vi "Run.vi"(8 "error in (no error)":errorcluster caption="entrée d'erreur (pas d'erreur)", 11 "Biclusters.lvclass":refnum<class "Biclusters.lvclass">) -> (0 "error out":errorcluster caption="sortie d'erreur", 2 "Data":T1, 3 "Biclusters.lvclass":refnum<class "Biclusters.lvclass">)   [LabVIEW 2020, in "Biclusters.lvclass"]
doc: "Returns : \n\nX : array of shape shape\n The generated array.\n\nrows : array of shape (n_clusters, X.shape[0],)\nThe indicators for cluster membership of each row.\n\ncols : array of shape (n_clusters, X.shape[1],)\nThe indicators for cluster membership of each column."
uses:
  Biclusters.lvclass
  Biclusters.lvclass/Biclusters.ctl
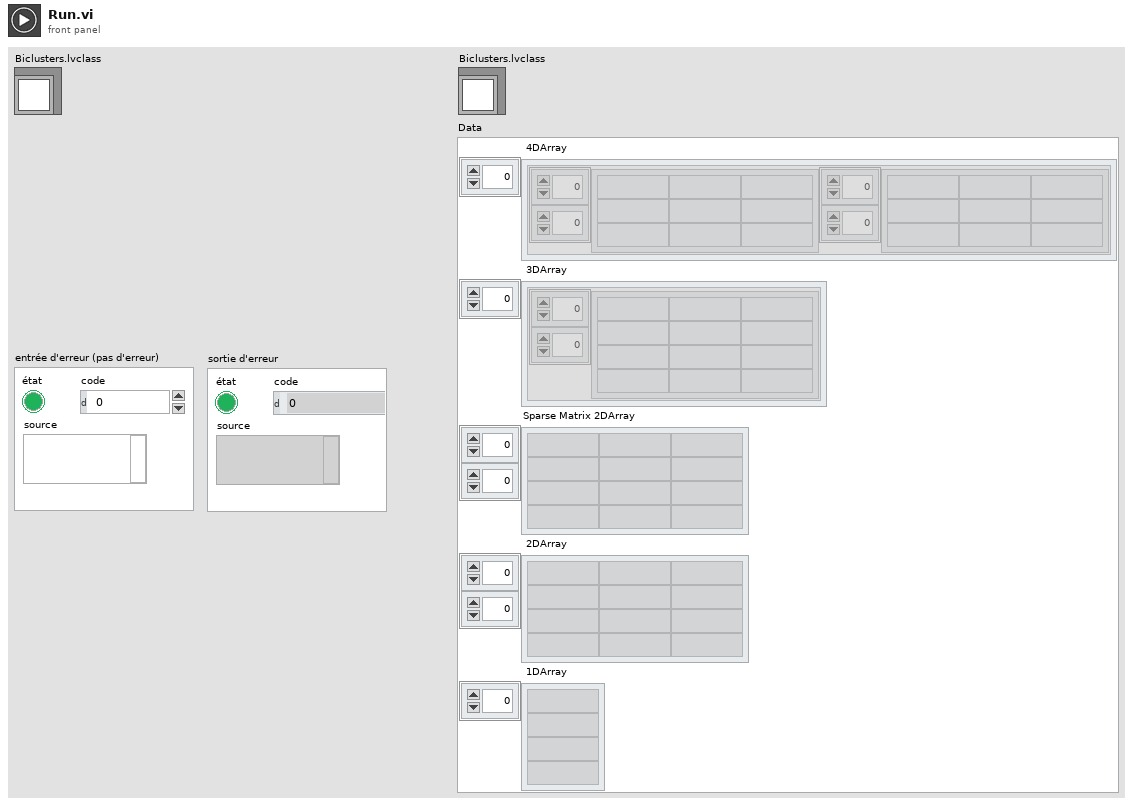
[diagram p1: front panel]
types:
  T1 = cluster{" 4DArray":cluster{"1":string[][], "2":string[][]}[], " 3DArray":cluster{"Tableau":string[][]}[], "Sparse Matrix 2DArray":string[][], " 2DArray":string[][], " 1DArray":string[]}
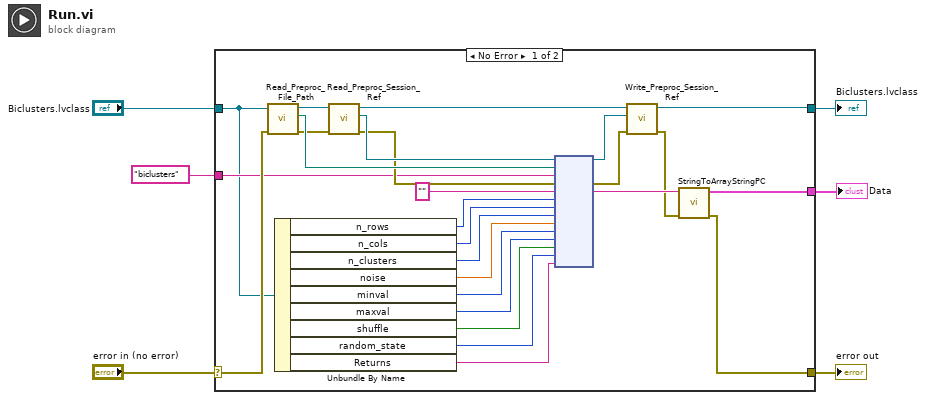
[diagram p0: block diagram]
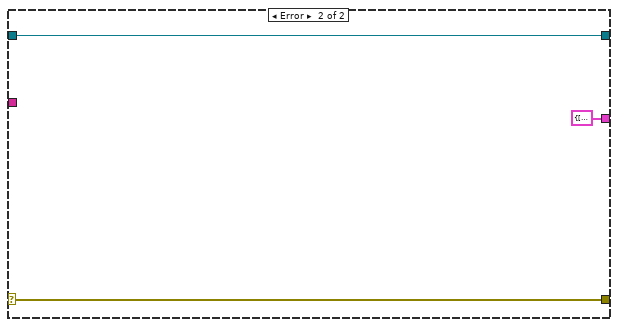
[diagram p2: hidden frame]
diagram:
  n1 = case shown="No Error" "error in (no error)" {
    selector: "error in (no error)" -> [w23 w35]
    tunnel: [w7 w35] -> w5
    tunnel: [w11 w34] -> w3
    tunnel: "Biclusters.lvclass" -> [w21 w34]
    tunnel: "biclusters" -> [w22 _]
    tunnel: [w9 T1 {" 4DArray"=[], " 3DArray"=[], "Sparse Matrix 2DArray"=[], " 2DArray"=[], " 1DArray"=[]} ("Data")] -> w1
    frame No Error {
      n2 = call-dynamic "Read_Preproc_File_Path.vi"("error in (no error)"=w23, "Python in"=w21) -> ("error out"=w27:errorcluster, "File_Path"=w30:path, "Python out"=w32:refnum<class "Biclusters.lvclass">)  [unwired: 7 in]
      n3 = Unbundle By Name(w21) -> ("n_rows"=w20:u32, "n_cols"=w19:u32, "n_clusters"=w18:u32, "noise"=w17:dbl, "minval"=w16:i32, "maxval"=w15:i32, "shuffle"=w14:bool, "random_state"=w13:i32, "Returns"=w12:string)
      n4 = call-dynamic "Read_Preproc_Session_Ref.vi"("error in (no error)"=w27, "Python in"=w32) -> ("error out"=w28:errorcluster, "Session_ref"=w29:refnum<k35>, "Python out"=w31:refnum<class "Biclusters.lvclass">)  [unwired: 7 in]
      n5 = node(w29, w30, w22, w28, "", w20, w19, w18, w17, w16, w15, w14, w13, w12) -> (w24:refnum<k35>, w26:errorcluster, w10:string)  [unwired: 9 in, 2 out]
      n6 = call-dynamic "Write_Preproc_Session_Ref.vi"("error in (no error)"=w26, "Session_ref"=w24, "Python in"=w31) -> ("error out"=w8:errorcluster, "Python out"=w11:refnum<class "Biclusters.lvclass">)  [unwired: 7 in]
      n7 = call "StringToArrayStringPC.vi"("sortie d'erreur"=w8, "Return value"=w10) -> ("sortie d'erreur"=w7:errorcluster, "Data"=w9:T1)  [unwired: 8 in]
    }
    frame Error {
    }
  }
  "error out" <- w5
  "Biclusters.lvclass" <- w3
  "Data" <- w1
